vi "trans全局.vi"() -> ()   [LabVIEW 2014]
panel:
  in  "distance":dbl[](array[numeric])
  in  "angle":dbl[](array[numeric])
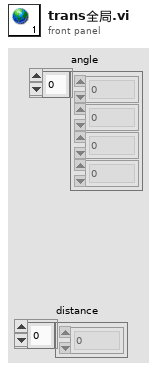
[diagram p1: front panel]
diagram:
